vi "Read SP_Set.vi"(8 "error in (no error)":errorcluster, 11 "Y_H in":refnum<class "Y_H.lvclass">) -> (0 "error out":errorcluster, 2 "SP_Set":dbl, 3 "Y_H out":refnum<class "Y_H.lvclass">)   [LabVIEW 2019, in "Y_H.lvclass"]
uses:
  Y_H.lvclass
  Y_H.lvclass/Y_H.ctl
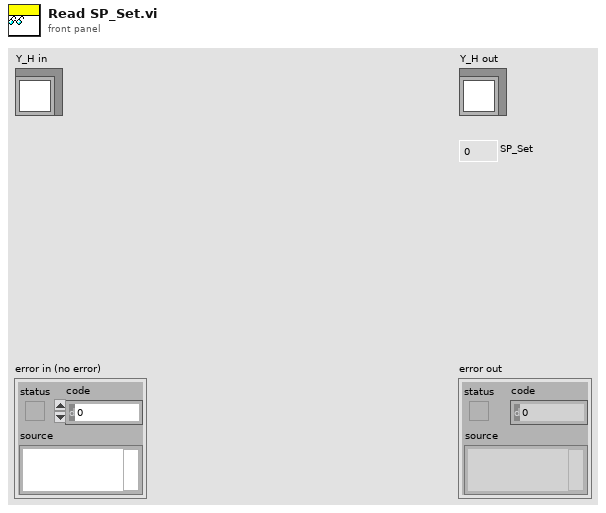
[diagram p1: front panel]
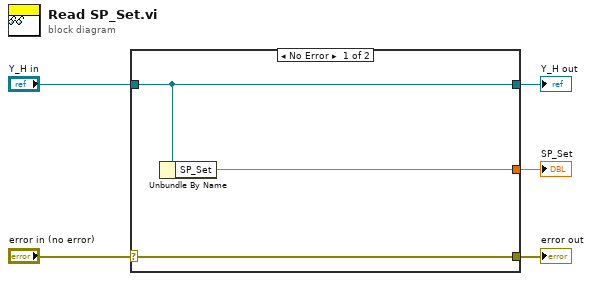
[diagram p0: block diagram]
diagram:
  n1 = case shown="No Error" "error in (no error)" {
    selector: "error in (no error)" -> [w8 w9]
    tunnel: [w8 w9] -> w4
    tunnel: [w7 w10] -> w2
    tunnel: "Y_H in" -> [w7 w10]
    tunnel: [w6 _] -> w1
    frame No Error {
      n2 = Unbundle By Name(w7) -> ("SP_Set"=w6:dbl)
    }
    frame Error {
    }
  }
  "error out" <- w4
  "Y_H out" <- w2
  "SP_Set" <- w1
